vi "save shape.vi"(8 "error in (no error)":errorcluster, 11 "BMC in":refnum<class "BMC.lvclass">) -> (0 "error out":errorcluster, 3 "BMC out":refnum<class "BMC.lvclass">)   [LabVIEW 2012, in "BMC.lvclass"]
uses:
  BMC.lvclass
  BMC.lvclass/BMC.ctl
  <vilib>/Utility/file.llb/Write To Spreadsheet File (DBL).vi
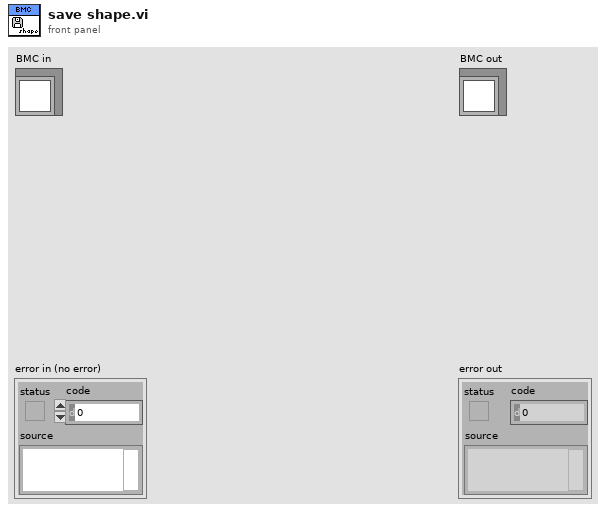
[diagram p1: front panel]
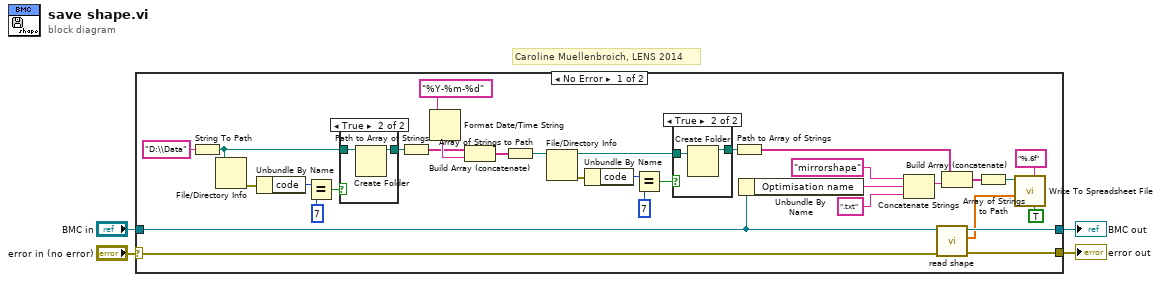
[diagram p0: block diagram]
diagram:
  # "Caroline Muellenbroich, LENS 2014"
  n1 = case shown="No Error" "error in (no error)" {
    selector: "error in (no error)" -> [w12 w44]
    tunnel: [w11 w44] -> w3
    tunnel: [w10 w43] -> w1
    tunnel: "BMC in" -> [w8 w43]
    frame No Error {
      n2 = String To Path(string="D:\\Data") -> (path=w17:path)
      n3 = File/Directory Info(path=w17) -> (error out=w13:errorcluster)  [unwired: 1 in, 6 out]
      n4 = Unbundle By Name(w13) -> ("code"=w14:i32)
      n5 = Equal?(x=w14, y=7) -> (x = y?=w16:bool)
      n6 = case shown="True" w16 {
        tunnel: w17 -> [w40 w42]
        tunnel: [w40 w41] -> w19
        frame False {
        }
        frame True {
          n7 = Create Folder(path (use dialog)=w42) -> (created path=w41:path)  [unwired: 1 in, 3 out]
        }
      }
      n8 = Path to Array of Strings(0:w19) -> (2:w21:string[])  [unwired: 1 out]
      n9 = Format Date/Time String(time format string (%c)="%Y-%m-%d") -> (date/time string=w22:string)  [unwired: 2 out]
      n10 = Build Array (concatenate)(w21, w22) -> (w23:string[])
      n11 = Array of Strings to Path(0:w23) -> (2:w25:path)  [unwired: 1 out]
      n12 = File/Directory Info(path=w25) -> (path out=w29:path, error out=w26:errorcluster)  [unwired: 1 in, 5 out]
      n13 = Unbundle By Name(w26) -> ("code"=w27:i32)
      n14 = Equal?(x=w27, y=7) -> (x = y?=w28:bool)
      n15 = case shown="True" w28 {
        tunnel: w29 -> [w37 w39]
        tunnel: [w37 w38] -> w34
        frame False {
        }
        frame True {
          n16 = Create Folder(path (use dialog)=w39) -> (created path=w38:path)  [unwired: 1 in, 3 out]
        }
      }
      n17 = Path to Array of Strings(0:w34) -> (2:w30:string[])  [unwired: 1 out]
      n18 = Unbundle By Name(w8) -> ("Optimisation name"=w7:string)
      n19 = Concatenate Strings("mirrorshape" ("string"), w7, ".txt" ("string")) -> (w31:string)
      n20 = call-dynamic "read shape.vi"("error in (no error)"=w12, "BMC in"=w8) -> ("error out"=w11:errorcluster, "1x160 Voltage Map"=w6:dbl[], "BMC out"=w10:refnum<class "BMC.lvclass">)  [unwired: 7 in]
      n21 = Build Array (concatenate)(w30, w31) -> (w32:string[])
      n22 = Array of Strings to Path(0:w32) -> (2:w9:path)  [unwired: 1 in]
      n23 = call-poly <vilib>:"Write To Spreadsheet File.vi"("transpose? (no:F)"=TRUE, "format (%.3f)"="%.6f", "1D data"=w6, "file path (dialog if empty)"=w9) -> ()  [unwired: 2 in, 3 out]
    }
    frame Error {
    }
  }
  "error out" <- w3
  "BMC out" <- w1
